vi "JSONtext Multi-step Filter.vi"() -> ()   [LabVIEW 2017] (continued)
\"ad\"\n    ],\n    \"friends\": [\n      {\n        \"id\": 0,\n        \"name\": \"Hayes Reynolds\"\n      },\n      {\n        \"id\": 1,\n        \"name\": \"Saundra Travis\"\n      },\n      {\n        \"id\": 2,\n        \"name\": \"Fuller Lucas\"\n      }\n    ],\n    \"greeting\": \"Hello, Alexander Jensen! You have 10 unread messages.\",\n    \"favoriteFruit\": \"apple\"\n  },\n  {\n    \"_id\": \"59b53bcb9eed49e2dc2bb115\",\n    \"index\": 53,\n    \"guid\": \"813e3bc6-1517-40ea-8506-03e41eb6ac3a\",\n    \"isActive\": true,\n    \"balance\": \"$1,392.46\",\n    \"picture\": \"http://placehold.it/32x32\",\n    \"age\": 33,\n    \"eyeColor\": \"green\",\n    \"name\": \"Rivas Rosales\",\n    \"gender\": \"male\",\n    \"company\": \"IPLAX\",\n    \"email\": \"rivasrosales@iplax.com\",\n    \"phone\": \"+1 (931) 434-2575\",\n    \"address\": \"124 Lake Avenue, Marysville, District Of Columbia, 5693\",\n    \"about\": \"Anim in duis adipisicing elit cupidatat aliqua tempor excepteur consectetur exercitation. Excepteur occaecat eiusmod incididunt anim sit in occaecat reprehenderit. Eu officia mollit ipsum aliquip adipisicing in ex consectetur enim Lorem irure pariatur irure ex. Ipsum nostrud labore commodo tempor. Occaecat ut sint tempor sunt anim nostrud nostrud excepteur duis aliqua consequat excepteur. Dolore ullamco enim irure magna anim nisi nostrud eiusmod proident.\\r\\n\",\n    \"registered\": \"2015-10-29T07:59:47 -00:00\",\n    \"latitude\": 35.539559,\n    \"longitude\": -171.582713,\n    \"tags\": [\n      \"qui\",\n      \"dolore\",\n      \"duis\",\n      \"nulla\",\n      \"est\",\n      \"ad\",\n      \"nulla\"\n    ],\n    \"friends\": [\n      {\n        \"id\": 0,\n        \"name\": \"Richard Chen\"\n      },\n      {\n        \"id\": 1,\n        \"name\": \"Pennington Garner\"\n      },\n      {\n        \"id\": 2,\n        \"name\": \"Ball Jackson\"\n      }\n    ],\n    \"greeting\": \"Hello, Rivas Rosales! You have 1 unread messages.\",\n    \"favoriteFruit\": \"apple\"\n  },\n  {\n    \"_id\": \"59b53bcb9e6f7027ee03d702\",\n    \"index\": 54,\n    \"guid\": \"577fde9f-2854-4414-9b96-06448ecb4488\",\n    \"isActive\": false,\n    \"balance\": \"$2,398.27\",\n    \"picture\": \"http://placehold.it/32x32\",\n    \"age\": 33,\n    \"eyeColor\": \"blue\",\n    \"name\": \"Jody Lancaster\",\n    \"gender\": \"female\",\n    \"company\": \"KEENGEN\",\n    \"email\": \"jodylancaster@keengen.com\",\n    \"phone\": \"+1 (898) 502-2640\",\n    \"address\": \"996 Quentin Street, Hoehne, Missouri, 4990\",\n    \"about\": \"Ipsum aute aute elit ea commodo amet laborum. Culpa quis reprehenderit proident consequat et enim. Adipisicing occaecat velit do labore eu eu id exercitation veniam ullamco elit. In ad Lorem ipsum proident enim. Tempor dolore Lorem et aute do excepteur dolore esse ad. Ut laboris pariatur elit officia anim consequat consequat officia eiusmod qui velit fugiat occaecat. Irure reprehenderit laborum cupidatat sint exercitation fugiat voluptate fugiat.\\r\\n\",\n    \"registered\": \"2015-08-06T02:13:32 -01:00\",\n    \"latitude\": 50.613083,\n    \"longitude\": 133.267848,\n    \"tags\": [\n      \"occaecat\",\n      \"dolore\",\n      \"quis\",\n      \"ullamco\",\n      \"ex\",\n      \"in\",\n      \"occaecat\"\n    ],\n    \"friends\": [\n      {\n        \"id\": 0,\n        \"name\": \"Barber Parks\"\n      },\n      {\n        \"id\": 1,\n        \"name\": \"Tamika Whitney\"\n      },\n      {\n        \"id\": 2,\n        \"name\": \"Boyle Melendez\"\n      }\n    ],\n    \"greeting\": \"Hello, Jody Lancaster! You have 6 unread messages.\",\n    \"favoriteFruit\": \"apple\"\n  },\n  {\n    \"_id\": \"59b53bcb218762e06bacfef0\",\n    \"index\": 55,\n    \"guid\": \"527e3426-cbe5-4fdc-ba02-0376d706325b\",\n    \"isActive\": true,\n    \"balance\": \"$2,126.86\",\n    \"picture\": \"http://placehold.it/32x32\",\n    \"age\": 22,\n    \"eyeColor\": \"brown\",\n    \"name\": \"Stout Lowe\",\n    \"gender\": \"male\",\n    \"company\": \"CHORIZON\",\n    \"email\": \"stoutlowe@chorizon.com\",\n    \"phone\": \"+1 (868) 502-2344\",\n    \"address\": \"228 Bliss Terrace, Loma, Illinois, 3866\",\n    \"about\": \"Nostrud et cillum nisi ea duis voluptate consequat excepteur labore laborum ut duis. Magna quis duis adipisicing duis elit nisi consequat duis laborum sint dolore. Esse adipisicing consectetur est esse amet ipsum Lorem aute incididunt amet. Enim est ea exercitation incididunt in.\\r\\n\",\n    \"registered\": \"2017-03-06T09:36:11 -00:00\",\n    \"latitude\": -33.017343,\n    \"longitude\": -113.928437,\n    \"tags\": [\n      \"labore\",\n      \"veniam\",\n      \"commodo\",\n      \"minim\",\n      \"qui\",\n      \"ad\",\n      \"et\"\n    ],\n    \"friends\": [\n      {\n        \"id\": 0,\n        \"name\": \"Trujillo Britt\"\n      },\n      {\n        \"id\": 1,\n        \"name\": \"Frye Moody\"\n      },\n      {\n        \"id\": 2,\n        \"name\": \"Gertrude Oneil\"\n      }\n    ],\n    \"greeting\": \"Hello, Stout Lowe! You have 1 unread messages.\",\n    \"favoriteFruit\": \"banana\"\n  },\n  {\n    \"_id\": \"59b53bcb16085e98ed2cea70\",\n    \"index\": 56,\n    \"guid\": \"3a610b27-0f08-447e-9216-39f2ad19273d\",\n    \"isActive\": true,\n    \"balance\": \"$1,799.97\",\n    \"picture\": \"http://placehold.it/32x32\",\n    \"age\": 38,\n    \"eyeColor\": \"brown\",\n    \"name\": \"Gwendolyn Farrell\",\n    \"gender\": \"female\",\n    \"company\": \"GEEKMOSIS\",\n    \"email\": \"gwendolynfarrell@geekmosis.com\",\n    \"phone\": \"+1 (807) 531-2875\",\n    \"address\": \"158 Chase Court, Riegelwood, Idaho, 6733\",\n    \"about\": \"Et Lorem reprehenderit aliqua pariatur velit dolor laboris fugiat. Consequat est dolor cillum consectetur cillum adipisicing laborum deserunt commodo non laboris. Non officia consequat consequat esse esse consequat. Eu fugiat minim ex deserunt.\\r\\n\",\n    \"registered\": \"2016-11-20T08:50:14 -00:00\",\n    \"latitude\": -38.469019,\n    \"longitude\": 102.32787,\n    \"tags\": [\n      \"ullamco\",\n      \"labore\",\n      \"dolor\",\n      \"consectetur\",\n      \"nisi\",\n      \"elit\",\n      \"cupidatat\"\n    ],\n    \"friends\": [\n      {\n        \"id\": 0,\n        \"name\": \"Blair Jordan\"\n      },\n      {\n        \"id\": 1,\n        \"name\": \"Wheeler Cannon\"\n      },\n      {\n        \"id\": 2,\n        \"name\": \"Dillon Fernandez\"\n      }\n    ],\n    \"greeting\": \"Hello, Gwendolyn Farrell! You have 4 unread messages.\",\n    \"favoriteFruit\": \"banana\"\n  },\n  {\n    \"_id\": \"59b53bcbd8b24e12c8941f72\",\n    \"index\": 57,\n    \"guid\": \"49be7373-8c53-4df1-9f56-ab81f211b8bf\",\n    \"isActive\": false,\n    \"balance\": \"$1,098.85\",\n    \"picture\": \"http://placehold.it/32x32\",\n    \"age\": 32,\n    \"eyeColor\": \"blue\",\n    \"name\": \"Gentry Anthony\",\n    \"gender\": \"male\",\n    \"company\": \"COGENTRY\",\n    \"email\": \"gentryanthony@cogentry.com\",\n    \"phone\": \"+1 (961) 457-3294\",\n    \"address\": \"807 Lewis Avenue, Aberdeen, Virgin Islands, 4388\",\n    \"about\": \"Qui cupidatat do veniam labore anim ullamco. Quis minim eu eiusmod labore consequat nulla labore. Est aliquip ut deserunt eiusmod occaecat laborum occaecat. Deserunt aliquip elit nostrud voluptate culpa magna occaecat non fugiat tempor labore elit cupidatat labore.\\r\\n\",\n    \"registered\": \"2016-04-30T03:18:07 -01:00\",\n    \"latitude\": 43.380138,\n    \"longitude\": -135.024374,\n    \"tags\": [\n      \"laboris\",\n      \"cillum\",\n      \"deserunt\",\n      \"excepteur\",\n      \"exercitation\",\n      \"do\",\n      \"tempor\"\n    ],\n    \"friends\": [\n      {\n        \"id\": 0,\n        \"name\": \"Janis Drake\"\n      },\n      {\n        \"id\": 1,\n        \"name\": \"Morse Huffman\"\n      },\n      {\n        \"id\": 2,\n        \"name\": \"Luna Davenport\"\n      }\n    ],\n    \"greeting\": \"Hello, Gentry Anthony! You have 7 unread messages.\",\n    \"favoriteFruit\": \"strawberry\"\n  },\n  {\n    \"_id\": \"59b53bcb21054f548ac53e2c\",\n    \"index\": 58,\n    \"guid\": \"efd6f059-3641-4df4-867c-58f72b8188dc\",\n    \"isActive\": false,\n    \"balance\": \"$3,534.32\",\n    \"picture\": \"http://placehold.it/32x32\",\n    \"age\": 26,\n    \"eyeColor\": \"brown\",\n    \"name\": \"Potter Hays\",\n    \"gender\": \"male\",\n    \"company\": \"ENTROFLEX\",\n    \"email\": \"potterhays@entroflex.com\",\n    \"phone\": \"+1 (905) 442-3818\",\n    \"address\": \"813 Erasmus Street, Northridge, Rhode Island, 5582\",\n    \"about\": \"Eiusmod Lorem laboris fugiat cupidatat qui dolore nulla nisi qui adipisicing. Cillum aute aliqua Lorem eiusmod. Ipsum sint eiusmod veniam pariatur excepteur officia consectetur deserunt. Cillum deserunt amet nostrud eiusmod deserunt labore nisi.\\r\\n\",\n    \"registered\": \"2017-05-24T04:37:42 -01:00\",\n    \"latitude\": 33.926864,\n    \"longitude\": -111.931141,\n    \"tags\": [\n      \"ipsum\",\n      \"commodo\",\n      \"dolor\",\n      \"nisi\",\n      \"dolore\",\n      \"laborum\",\n      \"incididunt\"\n    ],\n    \"friends\": [\n      {\n        \"id\": 0,\n        \"name\": \"Rosalie Livingston\"\n      },\n      {\n        \"id\": 1,\n        \"name\": \"Hannah Hardin\"\n      },\n      {\n        \"id\": 2,\n        \"name\": \"Madge Copeland\"\n      }\n    ],\n    \"greeting\": \"Hello, Potter Hays! You have 1 unread messages.\",\n    \"favoriteFruit\": \"apple\"\n  },\n  {\n    \"_id\": \"59b53bcbb0f4dd29011a5262\",\n    \"index\": 59,\n    \"guid\": \"530d5f1b-e3eb-49cc-8c7a-fc6f01b8ecdd\",\n    \"isActive\": false,\n    \"balance\": \"$3,138.39\",\n    \"picture\": \"http://placehold.it/32x32\",\n    \"age\": 20,\n    \"eyeColor\": \"blue\",\n    \"name\": \"Silvia Ortega\",\n    \"gender\": \"female\",\n    \"company\": \"CENTREXIN\",\n    \"email\": \"silviaortega@centrexin.com\",\n    \"phone\": \"+1 (980) 426-2287\",\n    \"address\": \"800 Williams Place, Chicopee, New Jersey, 3296\",\n    \"about\": \"Voluptate dolore do velit Lorem est voluptate ipsum aliquip ad officia exercitation laborum. Commodo consequat quis anim minim qui ut consectetur quis pariatur. Aute veniam sit Lorem voluptate esse amet. Esse cupidatat consequat cupidatat deserunt cillum magna ut reprehenderit esse non velit sint. Dolore nostrud ullamco ipsum culpa ad duis duis exercitation excepteur. Id consequat eu duis aliqua mollit.\\r\\n\",\n    \"registered\": \"2015-08-22T11:24:13 -01:00\",\n    \"latitude\": 81.63324,\n    \"longitude\": -118.965344,\n    \"tags\": [\n      \"laborum\",\n      \"excepteur\",\n      \"labore\",\n      \"ut\",\n      \"officia\",\n      \"in\",\n      \"eu\"\n    ],\n    \"friends\": [\n      {\n        \"id\": 0,\n        \"name\": \"Santiago Gentry\"\n      },\n      {\n        \"id\": 1,\n        \"name\": \"Melendez Pierce\"\n      },\n      {\n        \"id\": 2,\n        \"name\": \"Wood Stokes\"\n      }\n    ],\n    \"greeting\": \"Hello, Silvia Ortega! You have 8 unread messages.\",\n    \"favoriteFruit\": \"banana\"\n  },\n  {\n    \"_id\": \"59b53bcb2f824ae4587d2af7\",\n    \"index\": 60,\n    \"guid\": \"afe00138-7d3e-4a5b-9411-00d6155745e7\",\n    \"isActive\": true,\n    \"balance\": \"$2,759.26\",\n    \"picture\": \"http://placehold.it/32x32\",\n    \"age\": 34,\n    \"eyeColor\": \"green\",\n    \"name\": \"Combs Frazier\",\n    \"gender\": \"male\",\n    \"company\": \"ZIGGLES\",\n    \"email\": \"combsfrazier@ziggles.com\",\n    \"phone\": \"+1 (941) 567-3129\",\n    \"address\": \"154 Sedgwick Street, Elbert, Kentucky, 5956\",\n    \"about\": \"Anim incididunt dolor in eiusmod nulla do. Non consequat fugiat mollit laborum laborum occaecat nisi sunt Lorem consectetur laborum. Consequat laborum cupidatat dolore excepteur consequat adipisicing voluptate veniam aliquip elit do. Sint ut proident ex ea dolor aute fugiat et consequat minim pariatur do. Commodo laboris ea labore eiusmod labore fugiat consectetur enim. Cupidatat occaecat non minim dolor est commodo laborum excepteur anim. Eiusmod laboris laboris ullamco aliquip reprehenderit velit commodo aliqua magna anim irure non Lorem esse.\\r\\n\",\n    \"registered\": \"2016-07-23T05:27:36 -01:00\",\n    \"latitude\": -60.790167,\n    \"longitude\": -6.995975,\n    \"tags\": [\n      \"eu\",\n      \"irure\",\n      \"cupidatat\",\n      \"pariatur\",\n      \"sint\",\n      \"dolor\",\n      \"aliqua\"\n    ],\n    \"friends\": [\n      {\n        \"id\": 0,\n        \"name\": \"Karin Cortez\"\n      },\n      {\n        \"id\": 1,\n        \"name\": \"Ellen Ramos\"\n      },\n      {\n        \"id\": 2,\n        \"name\": \"Lynda Underwood\"\n      }\n    ],\n    \"greeting\": \"Hello, Combs Frazier! You have 6 unread messages.\",\n    \"favoriteFruit\": \"strawberry\"\n  },\n  {\n    \"_id\": \"59b53bcbebab6fc06e22bcf4\",\n    \"index\": 61,\n    \"guid\": \"30d1f10f-aad1-41f4-8621-5280977328d7\",\n    \"isActive\": true,\n    \"balance\": \"$2,802.02\",\n    \"picture\": \"http://placehold.it/32x32\",\n    \"age\": 33,\n    \"eyeColor\": \"blue\",\n    \"name\": \"Lyons Mccormick\",\n    \"gender\": \"male\",\n    \"company\": \"DECRATEX\",\n    \"email\": \"lyonsmccormick@decratex.com\",\n    \"phone\": \"+1 (978) 591-2593\",\n    \"address\": \"574 Kingsland Avenue, Calvary, Arizona, 2085\",\n    \"about\": \"Dolore cupidatat magna esse est est eiusmod non fugiat ipsum minim non duis do elit. Ut ad voluptate quis ea nostrud duis deserunt sit aliqua est sit consectetur. Aute eiusmod Lorem labore sint qui commodo. Quis quis ut minim ullamco. Nostrud in et enim sunt do voluptate qui nisi laborum non excepteur.\\r\\n\",\n    \"registered\": \"2014-08-18T12:17:12 -01:00\",\n    \"latitude\": 3.509991,\n    \"longitude\": -45.531481,\n    \"tags\": [\n      \"aliqua\",\n      \"culpa\",\n      \"et\",\n      \"eiusmod\",\n      \"nulla\",\n      \"esse\",\n      \"ad\"\n    ],\n    \"friends\": [\n      {\n        \"id\": 0,\n        \"name\": \"Rollins Owens\"\n      },\n      {\n        \"id\": 1,\n        \"name\": \"Erna Kim\"\n      },\n      {\n        \"id\": 2,\n        \"name\": \"Ferrell Blackburn\"\n      }\n    ],\n    \"greeting\": \"Hello, Lyons Mccormick! You have 3 unread messages.\",\n    \"favoriteFruit\": \"strawberry\"\n  },\n  {\n    \"_id\": \"59b53bcb4179085566efccff\",\n    \"index\": 62,\n    \"guid\": \"00011346-88e6-4501-9736-1458bea145f9\",\n    \"isActive\": false,\n    \"balance\": \"$3,659.33\",\n    \"picture\": \"http://placehold.it/32x32\",\n    \"age\": 40,\n    \"eyeColor\": \"green\",\n    \"name\": \"Cornelia Bray\",\n    \"gender\": \"female\",\n    \"company\": \"COMVEYER\",\n    \"email\": \"corneliabray@comveyer.com\",\n    \"phone\": \"+1 (959) 580-2744\",\n    \"address\": \"532 Butler Street, Crumpler, American Samoa, 8116\",\n    \"about\": \"Commodo commodo id amet minim labore mollit nulla et magna irure duis laboris. Culpa sunt Lorem eu cupidatat do aute nulla esse duis non velit incididunt commodo nulla. Pariatur in labore Lorem id in sit magna enim. Lorem Lorem exercitation velit sint do ullamco. Ipsum quis consequat elit nisi dolore ipsum. Non cillum est ad est sint nisi et. Reprehenderit tempor do minim ullamco consectetur.\\r\\n\",\n    \"registered\": \"2016-12-09T07:09:57 -00:00\",\n    \"latitude\": 2.702237,\n    \"longitude\": -80.758148,\n    \"tags\": [\n      \"cillum\",\n      \"excepteur\",\n      \"enim\",\n      \"amet\",\n      \"ipsum\",\n      \"mollit\",\n      \"dolore\"\n    ],\n    \"friends\": [\n      {\n        \"id\": 0,\n        \"name\": \"Hazel Steele\"\n      },\n      {\n        \"id\": 1,\n        \"name\": \"Beach Harmon\"\n      },\n      {\n        \"id\": 2,\n        \"name\": \"Olive Burton\"\n      }\n    ],\n    \"greeting\": \"Hello, Cornelia Bray! You have 7 unread messages.\",\n    \"favoriteFruit\": \"banana\"\n  },\n  {\n    \"_id\": \"59b53bcb3405dcede35b5a96\",\n    \"index\": 63,\n    \"guid\": \"db2142fc-3e37-4bd8-9c17-9891fe34a3b2\",\n    \"isActive\": true,\n    \"balance\": \"$1,405.92\",\n    \"picture\": \"http://placehold.it/32x32\",\n    \"age\": 36,\n    \"eyeColor\": \"brown\",\n    \"name\": \"Mcdonald Wade\",\n    \"gender\": \"male\",\n    \"company\": \"COMVERGES\",\n    \"email\": \"mcdonaldwade@comverges.com\",\n    \"phone\": \"+1 (937) 425-2339\",\n    \"address\": \"793 Elliott Walk, Waumandee, Massachusetts, 219\",\n    \"about\": \"Tempor irure minim proident adipisicing ad veniam magna minim nulla non sunt. Et eu ad non ea in occaecat irure dolore ex ipsum sunt. Adipisicing quis fugiat nostrud proident ullamco enim nostrud. Deserunt excepteur dolore anim sunt deserunt dolore non exercitation ex cupidatat eiusmod do. Tempor fugiat elit commodo id.\\r\\n\",\n    \"registered\": \"2015-04-21T01:38:34 -01:00\",\n    \"latitude\": -86.33219,\n    \"longitude\": -116.14479,\n    \"tags\": [\n      \"ex\",\n      \"in\",\n      \"et\",\n      \"est\",\n      \"officia\",\n      \"Lorem\",\n      \"qui\"\n    ],\n    \"friends\": [\n      {\n        \"id\": 0,\n        \"name\": \"Mariana Massey\"\n      },\n      {\n        \"id\": 1,\n        \"name\": \"Rosanne Strong\"\n      },\n      {\n        \"id\": 2,\n        \"name\": \"Fitzpatrick Riddle\"\n      }\n    ],\n    \"greeting\": \"Hello, Mcdonald Wade! You have 2 unread messages.\",\n    \"favoriteFruit\": \"apple\"\n  },\n  {\n    \"_id\": \"59b53bcb75995c65fa8a794e\",\n    \"index\": 64,\n    \"guid\": \"2d6b262c-1f4c-4818-8e0c-de99bc67de84\",\n    \"isActive\": false,\n    \"balance\": \"$3,597.88\",\n    \"picture\": \"http://placehold.it/32x32\",\n    \"age\": 20,\n    \"eyeColor\": \"green\",\n    \"name\": \"Leanne Briggs\",\n    \"gender\": \"female\",\n    \"company\": \"NAMEGEN\",\n    \"email\": \"leannebriggs@namegen.com\",\n    \"phone\": \"+1 (821) 566-2729\",\n    \"address\": \"126 Havens Place, Forbestown, Maine, 4804\",\n    \"about\": \"Exercitation sunt aliquip culpa cupidatat ad consectetur est dolor labore. Officia excepteur duis consectetur minim aliqua consectetur elit excepteur ipsum eiusmod aliquip mollit est. Incididunt pariatur id eiusmod nostrud nostrud Lorem culpa commodo fugiat officia ipsum aliquip. Reprehenderit aliquip irure ullamco proident elit minim ullamco sit pariatur dolore. Cillum voluptate anim amet cillum aliquip reprehenderit aliqua magna occaecat sit adipisicing laboris ea. Veniam aute dolore aliqua consectetur amet voluptate. Aliquip pariatur velit sit cillum nulla nostrud elit qui ipsum.\\r\\n\",\n    \"registered\": \"2017-01-31T02:36:59 -00:00\",\n    \"latitude\": -15.400663,\n    \"longitude\": 132.732197,\n    \"tags\": [\n      \"aute\",\n      \"quis\",\n      \"mollit\",\n      \"quis\",\n      \"pariatur\",\n      \"commodo\",\n      \"cupidatat\"\n    ],\n    \"friends\": [\n      {\n        \"id\": 0,\n        \"name\": \"Moran Curry\"\n      },\n      {\n        \"id\": 1,\n        \"name\": \"Mullins Ramsey\"\n      },\n      {\n        \"id\": 2,\n        \"name\": \"Pamela Perez\"\n      }\n    ],\n    \"greeting\": \"Hello, Leanne Briggs! You have 3 unread messages.\",\n    \"favoriteFruit\": \"banana\"\n  },\n  {\n    \"_id\": \"59b53bcbe6083b02455e297a\",\n    \"index\": 65,\n    \"guid\": \"114311fc-f902-4429-9713-509ccb6ad25e\",\n    \"isActive\": false,\n    \"balance\": \"$1,225.19\",\n    \"picture\": \"http://placehold.it/32x32\",\n    \"age\": 30,\n    \"eyeColor\": \"brown\",\n    \"name\": \"Lila Schmidt\",\n    \"gender\": \"female\",\n    \"company\": \"NEPTIDE\",\n    \"email\": \"lilaschmidt@neptide.com\",\n    \"phone\": \"+1 (904) 414-2477\",\n    \"address\": \"263 Degraw Street, Soham, Guam, 3945\",\n    \"about\": \"Anim culpa proident laboris non laboris. Velit nisi non nulla est Lorem laboris eu aliquip ex ea cupidatat aute nisi. Anim dolor sint pariatur cillum nisi nisi culpa. Fugiat velit non et anim non ex sint sint. Quis ex non labore commodo sit mollit eiusmod magna cillum laboris amet. Esse consequat qui velit et dolore pariatur id fugiat anim occaecat duis culpa in laborum.\\r\\n\",\n    \"registered\": \"2016-12-27T08:25:17 -00:00\",\n    \"latitude\": 21.703515,\n    \"longitude\": -54.394255,\n    \"tags\": [\n      \"incididunt\",\n      \"laboris\",\n      \"nulla\",\n      \"fugiat\",\n      \"aliquip\",\n      \"tempor\",\n      \"do\"\n    ],\n    \"friends\": [\n      {\n        \"id\": 0,\n        \"name\": \"Jordan Palmer\"\n      },\n      {\n        \"id\": 1,\n        \"name\": \"Leon Mcleod\"\n      },\n      {\n        \"id\": 2,\n        \"name\": \"Mcbride Simon\"\n      }\n    ],\n    \"greeting\": \"Hello, Lila Schmidt! You have 5 unread messages.\",\n    \"favoriteFruit\": \"strawberry\"\n  },\n  {\n    \"_id\": \"59b53bcb48e4a6fa9e53affd\",\n    \"index\": 66,\n    \"guid\": \"34a3b2a0-9e97-4dab-881d-bc809370ed0b\",\n    \"isActive\": true,\n    \"balance\": \"$2,539.75\",\n    \"picture\": \"http://placehold.it/32x32\",\n    \"age\": 38,\n    \"eyeColor\": \"green\",\n    \"name\": \"Melba House\",\n    \"gender\": \"female\",\n    \"company\": \"NETUR\",\n    \"email\": \"melbahouse@netur.com\",\n    \"phone\": \"+1 (975) 559-3215\",\n    \"address\": \"688 Tillary Street, Ruffin, Texas, 920\",\n    \"about\": \"Ad non aliquip tempor aute ea anim cillum officia qui proident esse culpa reprehenderit. Consectetur eiusmod quis velit sint dolore est velit voluptate laboris sunt occaecat consectetur consectetur ipsum. Proident sint elit dolor amet occaecat. Dolore reprehenderit consectetur commodo mollit pariatur aliqua magna fugiat nostrud cupidatat. Nostrud do esse laboris ipsum ullamco dolore officia. Ut labore elit non labore aute magna pariatur laborum ullamco velit laborum duis elit do. Ullamco labore nulla eiusmod sint.\\r\\n\",\n    \"registered\": \"2016-04-17T08:18:11 -01:00\",\n    \"latitude\": 87.963824,\n    \"longitude\": 65.388805,\n    \"tags\": [\n      \"est\",\n      \"cillum\",\n      \"veniam\",\n      \"exercitation\",\n      \"aliqua\",\n      \"velit\",\n      \"nulla\"\n    ],\n    \"friends\": [\n      {\n        \"id\": 0,\n        \"name\": \"Erica Moran\"\n      },\n      {\n        \"id\": 1,\n        \"name\": \"Peck Rios\"\n      },\n      {\n        \"id\": 2,\n        \"name\": \"Irene Wiley\"\n      }\n    ],\n    \"greeting\": \"Hello, Melba House! You have 3 unread messages.\",\n    \"favoriteFruit\": \"banana\"\n  },\n  {\n    \"_id\": \"59b53bcb23c882b00ccbeb78\",\n    \"index\": 67,\n    \"guid\": \"43870cc3-e38d-40e7-ba96-33fff3de9315\",\n    \"isActive\": false,\n    \"balance\": \"$2,394.68\",\n    \"picture\": \"http://placehold.it/32x32\",\n    \"age\": 20,\n    \"eyeColor\": \"brown\",\n    \"name\": \"Vance Thompson\",\n    \"gender\": \"male\",\n    \"company\": \"BIOSPAN\",\n    \"email\": \"vancethompson@biospan.com\",\n    \"phone\": \"+1 (930) 463-3961\",\n    \"address\": \"573 Dearborn Court, Jacumba, Colorado, 1903\",\n    \"about\": \"Duis aliquip aliquip ut pariatur cupidatat magna enim qui. Culpa tempor laboris et culpa eiusmod. Aute excepteur nulla ullamco nulla aute cillum laborum irure eiusmod. Id exercitation nostrud veniam elit eu excepteur quis id ad. Aute velit sit nulla incididunt amet consectetur anim.\\r\\n\",\n    \"registered\": \"2015-01-06T09:28:15 -00:00\",\n    \"latitude\": 16.206121,\n    \"longitude\": 2.066817,\n    \"tags\": [\n      \"proident\",\n      \"officia\",\n      \"do\",\n      \"irure\",\n      \"qui\",\n      \"sint\",\n      \"consequat\"\n    ],\n    \"friends\": [\n      {\n        \"id\": 0,\n        \"name\": \"Marilyn Justice\"\n      },\n      {\n        \"id\": 1,\n        \"name\": \"Pacheco Frank\"\n      },\n      {\n        \"id\": 2,\n        \"name\": \"Warner Neal\"\n      }\n    ],\n    \"greeting\": \"Hello, Vance Thompson! You have 8 unread messages.\",\n    \"favoriteFruit\": \"banana\"\n  },\n  {\n    \"_id\": \"59b53bcb41a2c54c5e49f6e2\",\n    \"index\": 68,\n    \"guid\": \"f0ac1d16-e1c6-4208-8964-a7f523b09527\",\n    \"isActive\": false,\n    \"balance\": \"$2,631.00\",\n    \"picture\": \"http://placehold.it/32x32\",\n    \"age\": 36,\n    \"eyeColor\": \"brown\",\n    \"name\": \"Burton Dorsey\",\n    \"gender\": \"male\",\n    \"company\": \"ROTODYNE\",\n    \"email\": \"burtondorsey@rotodyne.com\",\n    \"phone\": \"+1 (824) 463-3076\",\n    \"address\": \"914 Belmont Avenue, Takilma, Utah, 4995\",\n    \"about\": \"Fugiat irure proident quis duis laborum occaecat. Irure voluptate deserunt dolor reprehenderit do anim deserunt adipisicing. Ex in quis eu irure qui laborum duis do occaecat. Reprehenderit commodo commodo officia do incididunt velit ipsum. Voluptate elit ullamco cupidatat enim duis magna consequat ipsum mollit.\\r\\n\",\n    \"registered\": \"2015-06-21T09:38:28 -01:00\",\n    \"latitude\": 29.679351,\n    \"longitude\": 55.009156,\n    \"tags\": [\n      \"id\",\n      \"anim\",\n      \"do\",\n      \"eiusmod\",\n      \"sunt\",\n      \"dolor\",\n      \"ullamco\"\n    ],\n    \"friends\": [\n      {\n        \"id\": 0,\n        \"name\": \"Estrada Frederick\"\n      },\n      {\n        \"id\": 1,\n        \"name\": \"Pratt Bernard\"\n      },\n      {\n        \"id\": 2,\n        \"name\": \"Bobbie Pope\"\n      }\n    ],\n    \"greeting\": \"Hello, Burton Dorsey! You have 1 unread messages.\",\n    \"favoriteFruit\": \"apple\"\n  },\n  {\n    \"_id\": \"59b53bcbd77a0c5752db5b53\",\n    \"index\": 69,\n    \"guid\": \"9c501418-7230-4ccb-832a-d344a905dd2d\",\n    \"isActive\": true,\n    \"balance\": \"$3,815.52\",\n    \"picture\": \"http://placehold.it/32x32\",\n    \"age\": 27,\n    \"eyeColor\": \"brown\",\n    \"name\": \"Hatfield Ball\",\n    \"gender\": \"male\",\n    \"company\": \"ZINCA\",\n    \"email\": \"hatfieldball@zinca.com\",\n    \"phone\": \"+1 (989) 422-3125\",\n    \"address\": \"768 Guernsey Street, Brewster, Montana, 139\",\n    \"about\": \"Aute eiusmod eu nisi ut cupidatat. Duis minim sunt amet labore. Ullamco nisi Lorem ipsum qui anim id laboris incididunt excepteur id culpa sit excepteur dolore. Nulla eu excepteur do id quis. Ullamco culpa cupidatat culpa non aliquip tempor duis ad et sunt minim consectetur. Aliquip sit aliqua nisi sunt elit ea.\\r\\n\",\n    \"registered\": \"2014-06-10T12:39:52 -01:00\",\n    \"latitude\": 56.126846,\n    \"longitude\": 40.545126,\n    \"tags\": [\n      \"amet\",\n      \"veniam\",\n      \"dolor\",\n      \"in\",\n      \"excepteur\",\n      \"nulla\",\n      \"qui\"\n    ],\n    \"friends\": [\n      {\n        \"id\": 0,\n        \"name\": \"Stewart Peterson\"\n      },\n      {\n        \"id\": 1,\n        \"name\": \"Heather Mayo\"\n      },\n      {\n        \"id\": 2,\n        \"name\": \"Murray Brady\"\n      }\n    ],\n    \"greeting\": \"Hello, Hatfield Ball! You have 8 unread messages.\",\n    \"favoriteFruit\": \"apple\"\n  },\n  {\n    \"_id\": \"59b53bcb1fec7ace6110275b\",\n    \"index\": 70,\n    \"guid\": \"f7def176-2ac0-4c08-b1dc-d51a5a67dc0b\",\n    \"isActive\": true,\n    \"balance\": \"$2,019.28\",\n    \"picture\": \"http://placehold.it/32x32\",\n    \"age\": 22,\n    \"eyeColor\": \"blue\",\n    \"name\": \"Hill Shelton\",\n    \"gender\": \"male\",\n    \"company\": \"EMTRAK\",\n    \"email\": \"hillshelton@emtrak.com\",\n    \"phone\": \"+1 (868) 415-2186\",\n    \"address\": \"231 Loring Avenue, Jeff, Maryland, 4988\",\n    \"about\": \"Veniam id eu deserunt laborum. Veniam labore anim amet sunt officia ea cupidatat deserunt. Aute proident commodo est mollit amet laborum dolore pariatur culpa. Ad adipisicing ea laboris excepteur ex id est magna reprehenderit. Excepteur aliqua do commodo cupidatat velit do.\\r\\n\",\n    \"registered\": \"2016-09-29T01:14:11 -01:00\",\n    \"latitude\": 9.893931,\n    \"longitude\": 1.018174,\n    \"tags\": [\n      \"anim\",\n      \"fugiat\",\n      \"culpa\",\n      \"mollit\",\n      \"do\",\n      \"voluptate\",\n      \"consequat\"\n    ],\n    \"friends\": [\n      {\n        \"id\": 0,\n        \"name\": \"Glass Walter\"\n      },\n      {\n        \"id\": 1,\n        \"name\": \"Joyce Church\"\n      },\n      {\n        \"id\": 2,\n        \"name\": \"Kari Bowen\"\n      }\n    ],\n    \"greeting\": \"Hello, Hill Shelton! You have 8 unread messages.\",\n    \"favoriteFruit\": \"apple\"\n  },\n  {\n    \"_id\": \"59b53bcb0018db268644035f\",\n    \"index\": 71,\n    \"guid\": \"892c26d8-1618-4249-a5cd-2e4f72a42917\",\n    \"isActive\": true,\n    \"balance\": \"$3,320.73\",\n    \"picture\": \"http://placehold.it/32x32\",\n    \"age\": 22,\n    \"eyeColor\": \"brown\",\n    \"name\": \"Jamie Curtis\",\n    \"gender\": \"female\",\n    \"company\": \"OPTICON\",\n    \"email\": \"jamiecurtis@opticon.com\",\n    \"phone\": \"+1 (987) 560-2955\",\n    \"address\": \"798 Woodpoint Road, Zarephath, Connecticut, 258\",\n    \"about\": \"Occaecat duis commodo et eiusmod amet. Et minim aliqua commodo ipsum dolore cupidatat aute quis sint ullamco laborum. Culpa consequat dolor sunt mollit magna ad nisi cillum aliqua eu veniam nostrud. Velit tempor consequat culpa et irure. Aute culpa duis cupidatat nulla ut et incididunt officia magna irure enim do esse.\\r\\n\",\n    \"registered\": \"2016-05-17T11:58:35 -01:00\",\n    \"latitude\": -25.764923,\n    \"longitude\": 176.326556,\n    \"tags\": [\n      \"veniam\",\n      \"reprehenderit\",\n      \"reprehenderit\",\n      \"sunt\",\n      \"ea\",\n      \"non\",\n      \"veniam\"\n    ],\n    \"friends\": [\n      {\n        \"id\": 0,\n        \"name\": \"Katy Mccoy\"\n      },\n      {\n        \"id\": 1,\n        \"name\": \"Marianne Merrill\"\n      },\n      {\n        \"id\": 2,\n        \"name\": \"Bass Pugh\"\n      }\n    ],\n    \"greeting\": \"Hello, Jamie Curtis! You have 3 unread messages.\",\n    \"favoriteFruit\": \"apple\"\n  },\n  {\n    \"_id\": \"59b53bcb66c0788939f5655d\",\n    \"index\": 72,\n    \"guid\": \"2d7d871b-187c-4eea-9abc-7d1b4a70dd40\",\n    \"isActive\": false,\n    \"balance\": \"$1,923.95\",\n    \"picture\": \"http://placehold.it/32x32\",\n    \"age\": 35,\n    \"eyeColor\": \"brown\",\n    \"name\": \"Wanda Cote\",\n    \"gender\": \"female\",\n    \"company\": \"RONBERT\",\n    \"email\": \"wandacote@ronbert.com\",\n    \"phone\": \"+1 (953) 577-2066\",\n    \"address\": \"352 Louisiana Avenue, Wadsworth, Iowa, 354\",\n    \"about\": \"Qui ad duis consequat Lorem et nisi fugiat non et deserunt pariatur. Ullamco et velit aute magna officia ullamco culpa. Laborum pariatur ex deserunt laborum.\\r\\n\",\n    \"registered\": \"2016-07-05T06:46:18 -01:00\",\n    \"latitude\": 74.488765,\n    \"longitude\": 47.891038,\n    \"tags\": [\n      \"adipisicing\",\n      \"anim\",\n      \"sit\",\n      \"quis\",\n      \"ipsum\",\n      \"aliqua\",\n      \"officia\"\n    ],\n    \"friends\": [\n      {\n        \"id\": 0,\n        \"name\": \"Heath Joseph\"\n      },\n      {\n        \"id\": 1,\n        \"name\": \"Manning Jarvis\"\n      },\n      {\n        \"id\": 2,\n        \"name\": \"Wall Heath\"\n      }\n    ],\n    \"greeting\": \"Hello, Wanda Cote! You have 8 unread messages.\",\n    \"favoriteFruit\": \"apple\"\n  },\n  {\n    \"_id\": \"59b53bcb084c37005beb12b0\",\n    \"index\": 73,\n    \"guid\": \"b7330764-4c34-40a3-9958-195fab4b3d91\",\n    \"isActive\": false,\n    \"balance\": \"$2,499.95\",\n    \"picture\": \"http://placehold.it/32x32\",\n    \"age\": 29,\n    \"eyeColor\": \"blue\",\n    \"name\": \"Herman Parsons\",\n    \"gender\": \"male\",\n    \"company\": \"CANOPOLY\",\n    \"email\": \"hermanparsons@canopoly.com\",\n    \"phone\": \"+1 (858) 469-2039\",\n    \"address\": \"406 Ingraham Street, Freeburn, Wyoming, 9051\",\n    \"about\": \"Officia fugiat voluptate dolore ut ex elit. Proident non sint culpa incididunt ipsum aliquip occaecat dolore. Non enim anim aute consectetur in ex. Pariatur sint labore anim non dolor duis amet nisi cupidatat sit laborum anim veniam eiusmod. Do veniam voluptate eiusmod irure eiusmod ullamco veniam adipisicing laborum est laborum aliquip. Deserunt ex in magna eu aute excepteur ea. Excepteur ipsum aliquip nostrud anim.\\r\\n\",\n    \"registered\": \"2016-03-18T07:09:45 -00:00\",\n    \"latitude\": 45.260943,\n    \"longitude\": 94.785454,\n    \"tags\": [\n      \"nisi\",\n      \"ipsum\",\n      \"esse\",\n      \"culpa\",\n      \"dolore\",\n      \"elit\",\n      \"in\"\n    ],\n    \"friends\": [\n      {\n        \"id\": 0,\n        \"name\": \"Walsh Mcdaniel\"\n      },\n      {\n        \"id\": 1,\n        \"name\": \"Hardin Carter\"\n      },\n      {\n        \"id\": 2,\n        \"name\": \"Stuart Hall\"\n      }\n    ],\n    \"greeting\": \"Hello, Herman Parsons! You have 8 unread messages.\",\n    \"favoriteFruit\": \"banana\"\n  },\n  {\n    \"_id\": \"59b53bcb527263f7fc30c523\",\n    \"index\": 74,\n    \"guid\": \"61ea1af5-38ec-49ca-a918-8c9be1df0919\",\n    \"isActive\": true,\n    \"balance\": \"$2,336.60\",\n    \"picture\": \"http://placehold.it/32x32\",\n    \"age\": 36,\n    \"eyeColor\": \"brown\",\n    \"name\": \"Patterson Benton\",\n    \"gender\": \"male\",\n    \"company\": \"UTARIAN\",\n    \"email\": \"pattersonbenton@utarian.com\",\n    \"phone\": \"+1 (976) 509-3593\",\n    \"address\": \"459 Hampton Place, Leola, Marshall Islands, 109\",\n    \"about\": \"Cupidatat do anim deserunt enim. Sint id consectetur culpa consectetur duis ex occaecat eiusmod eu mollit ipsum minim. Sint incididunt aliqua velit in. Aliquip eiusmod esse ad est aute laborum est sunt ea esse. Quis eu deserunt aute pariatur qui. Proident incididunt nisi id mollit et dolor veniam adipisicing aliqua eu excepteur id sint exercitation.\\r\\n\",\n    \"registered\": \"2016-09-11T07:59:11 -01:00\",\n    \"latitude\": -34.270598,\n    \"longitude\": 173.169207,\n    \"tags\": [\n      \"voluptate\",\n      \"consectetur\",\n      \"voluptate\",\n      \"fugiat\",\n      \"laboris\",\n      \"cillum\",\n      \"occaecat\"\n    ],\n    \"friends\": [\n      {\n        \"id\": 0,\n        \"name\": \"Campbell Swanson\"\n      },\n      {\n        \"id\": 1,\n        \"name\": \"Jenkins Fuller\"\n      },\n      {\n        \"id\": 2,\n        \"name\": \"Boyer Maxwell\"\n      }\n    ],\n    \"greeting\": \"Hello, Patterson Benton! You have 3 unread messages.\",\n    \"favoriteFruit\": \"banana\"\n  },\n  {\n    \"_id\": \"59b53bcb55cf0122e1804227\",\n    \"index\": 75,\n    \"guid\": \"6410aae3-9791-4171-bc46-fe1160c2d3d4\",\n    \"isActive\": false,\n    \"balance\": \"$2,752.83\",\n    \"picture\": \"http://placehold.it/32x32\",\n    \"age\": 31,\n    \"eyeColor\": \"green\",\n    \"name\": \"Gracie Luna\",\n    \"gender\": \"female\",\n    \"company\": \"NEWCUBE\",\n    \"email\": \"gracieluna@newcube.com\",\n    \"phone\": \"+1 (950) 514-3889\",\n    \"address\": \"112 Arlington Place, Alfarata, Nevada, 8390\",\n    \"about\": \"Quis amet amet proident magna aliqua pariatur id cupidatat. Et duis ipsum eiusmod exercitation cillum voluptate voluptate cupidatat veniam elit veniam culpa. Eiusmod excepteur proident est in occaecat. Cillum veniam eiusmod laboris irure qui nostrud sit duis ullamco. Nostrud ullamco sint ad esse laborum consectetur anim aliquip ea veniam voluptate in. Adipisicing tempor ea pariatur ex nisi deserunt nostrud duis. Quis pariatur in deserunt Lorem laborum laborum.\\r\\n\",\n    \"registered\": \"2016-01-24T04:20:49 -00:00\",\n    \"latitude\": 65.338318,\n    \"longitude\": -113.569985,\n    \"tags\": [\n      \"Lorem\",\n      \"proident\",\n      \"pariatur\",\n      \"nisi\",\n      \"ex\",\n      \"sit\",\n      \"minim\"\n    ],\n    \"friends\": [\n      {\n        \"id\": 0,\n        \"name\": \"Marshall Whitaker\"\n      },\n      {\n        \"id\": 1,\n        \"name\": \"Franco Randolph\"\n      },\n      {\n        \"id\": 2,\n        \"name\": \"Rodgers Acevedo\"\n      }\n    ],\n    \"greeting\": \"Hello, Gracie Luna! You have 2 unread messages.\",\n    \"favoriteFruit\": \"banana\"\n  },\n  {\n    \"_id\": \"59b53bcb8af5d0cb60390e81\",\n    \"index\": 76,\n    \"guid\": \"e3634b1c-9b8a-4352-811b-26ea270eb854\",\n    \"isActive\": true,\n    \"balance\": \"$2,462.40\",\n    \"picture\": \"http://placehold.it/32x32\",\n    \"age\": 39,\n    \"eyeColor\": \"blue\",\n    \"name\": \"Landry Townsend\",\n    \"gender\": \"male\",\n    \"company\": \"COMTRACT\",\n    \"email\": \"landrytownsend@comtract.com\",\n    \"phone\": \"+1 (904) 551-3761\",\n    \"address\": \"223 Rockwell Place, Coalmont, North Carolina, 9268\",\n    \"about\": \"Dolore ipsum occaecat quis deserunt excepteur consequat officia sit elit ea deserunt deserunt ut velit. Magna cupidatat dolore velit duis ullamco cupidatat eu fugiat do sint cupidatat dolore. In qui amet occaecat nisi consectetur consectetur ipsum aliquip excepteur nostrud ut quis fugiat dolor. Fugiat eu proident proident fugiat enim anim cupidatat elit sint consectetur irure est eu.\\r\\n\",\n    \"registered\": \"2015-12-01T12:13:22 -00:00\",\n    \"latitude\": 26.684426,\n    \"longitude\": 37.304822,\n    \"tags\": [\n      \"reprehenderit\",\n      \"officia\",\n      \"ad\",\n      \"Lorem\",\n      \"proident\",\n      \"amet\",\n      \"minim\"\n    ],\n    \"friends\": [\n      {\n        \"id\": 0,\n        \"name\": \"Tommie Hayes\"\n      },\n      {\n        \"id\": 1,\n        \"name\": \"Ana Morgan\"\n      },\n      {\n        \"id\": 2,\n        \"name\": \"Snow Sherman\"\n      }\n    ],\n    \"greeting\": \"Hello, Landry Townsend! You have 4 unread messages.\",\n    \"favoriteFruit\": \"banana\"\n  },\n  {\n    \"_id\": \"59b53bcb2c27fefc63f2a7ae\",\n    \"index\": 77,\n    \"guid\": \"88476412-4c1a-4f8f-994a-6d052651dcd4\",\n    \"isActive\": true,\n    \"balance\": \"$1,302.88\",\n    \"picture\": \"http://placehold.it/32x32\",\n    \"age\": 36,\n    \"eyeColor\": \"blue\",\n    \"name\": \"Janelle Patton\",\n    \"gender\": \"female\",\n    \"company\": \"QUAREX\",\n    \"email\": \"janellepatton@quarex.com\",\n    \"phone\": \"+1 (913) 416-3894\",\n    \"address\": \"890 Waldane Court, Clinton, New Mexico, 861\",\n    \"about\": \"Pariatur deserunt Lorem magna aliquip ea esse aliqua irure. Esse eiusmod esse excepteur et sit proident cupidatat adipisicing officia et fugiat. Et esse eiusmod laboris aute est elit. Incididunt consequat et irure cupidatat incididunt qui reprehenderit aliqua in. Labore aliqua qui amet elit. Magna in exercitation incididunt esse fugiat deserunt deserunt Lorem tempor. Et pariatur pariatur incididunt labore ut occaecat laboris pariatur pariatur.\\r\\n\",\n    \"registered\": \"2015-06-17T10:19:36 -01:00\",\n    \"latitude\": -46.295286,\n    \"longitude\": 176.279204,\n    \"tags\": [\n      \"do\",\n      \"reprehenderit\",\n      \"voluptate\",\n      \"ullamco\",\n      \"duis\",\n      \"do\",\n      \"culpa\"\n    ],\n    \"friends\": [\n      {\n        \"id\": 0,\n        \"name\": \"Brandy Dalton\"\n      },\n      {\n        \"id\": 1,\n        \"name\": \"Norris Sparks\"\n      },\n      {\n        \"id\": 2,\n        \"name\": \"Cobb Dyer\"\n      }\n    ],\n    \"greeting\": \"Hello, Janelle Patton! You have 8 unread messages.\",\n    \"favoriteFruit\": \"apple\"\n  },\n  {\n    \"_id\": \"59b53bcbeaa09930d8cb67e3\",\n    \"index\": 78,\n    \"guid\": \"aa15604b-5a80-4a46-ac58-e1f7b908819a\",\n    \"isActive\": false,\n    \"balance\": \"$3,040.74\",\n    \"picture\": \"http://placehold.it/32x32\",\n    \"age\": 30,\n    \"eyeColor\": \"blue\",\n    \"name\": \"Agnes Frye\",\n    \"gender\": \"female\",\n    \"company\": \"SARASONIC\",\n    \"email\": \"agnesfrye@sarasonic.com\",\n    \"phone\": \"+1 (883) 528-2733\",\n    \"address\": \"798 Evans Street, Freelandville, Michigan, 1541\",\n    \"about\": \"Aliqua veniam ullamco nisi amet. Officia in anim minim amet minim cupidatat esse 
